vi "Update.vi"(8 "error in (no error)":errorcluster, 10 "Message in":refnum<class "UpdateMessage.lvclass">, 11 "Piezo in":refnum<class "Piezo.lvclass">) -> (0 "error out":errorcluster, 3 "Piezo out":refnum<class "Piezo.lvclass">)   [LabVIEW 2012, in "Piezo.lvclass"]
doc: "The update method processes the command 'update'. \n\nThe command 'update' is used for receiving new values to be set to the private data of the class. This could be seen as a public set method for setting new parameters to the private class data."
uses:
  Piezo.lvclass
  <vilib>/Distrio/Murmex/UpdateMessage/UpdateMessage.lvclass
  <vilib>/Distrio/Murmex/Murmex/Murmex.lvclass
panel:
  # "This method is called when the UPDATE\ntrigger is sent. \n\nOverride this method when your component needs to\nrespond to this trigger. \n\nCall parent for proper implementation"
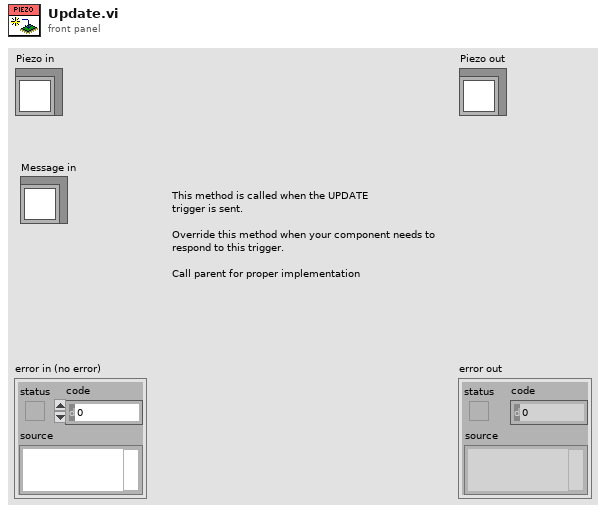
[diagram p1: front panel]
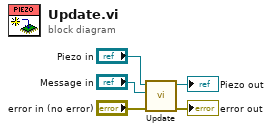
[diagram p0: block diagram]
diagram:
  n1 = call-parent "Update.vi"("error in (no error)"="error in (no error)", "Message in"="Message in", "Murmex in"="Piezo in") -> ("error out"=→"error out":errorcluster, "Murmex out"=→"Piezo out":refnum<class "Piezo.lvclass">)  [unwired: 7 in]
